vi "DAQ-WriteArray.vi"(4 "DAQ?":bool, 5 "Control Array":dbl[](array[numeric]), 6 "Limites":T2, 7 "#samples":u32, 8 "DAQ Device IN":T1={"DAQ Fs (S/s)"=10000.0, "task"="", "error"={"status"=FALSE, "code"=0, "source"=""}, "Min Value"=-10.0, "Max Value"=10.0}) -> (0 "Waveform Graph":waveform(dbl)(graph), 3 "DAQ Device OUT":T1={"DAQ Fs (S/s)"=0.0, "task"="", "error"={"status"=FALSE, "code"=0, "source"=""}, "Min Value"=-10.0, "Max Value"=10.0})   [LabVIEW 2010]
uses:
  <vilib>/DAQmx/write.llb/DAQmx Write (Analog Wfm 1Chan NSamp).vi
  <vilib>/daqmx/miscellaneous.llb/DAQmx Fill In Error Info.vi
panel:
  out "#samples 2":u32
  out "#samples out":u32
  out "Waveform":waveform(dbl)
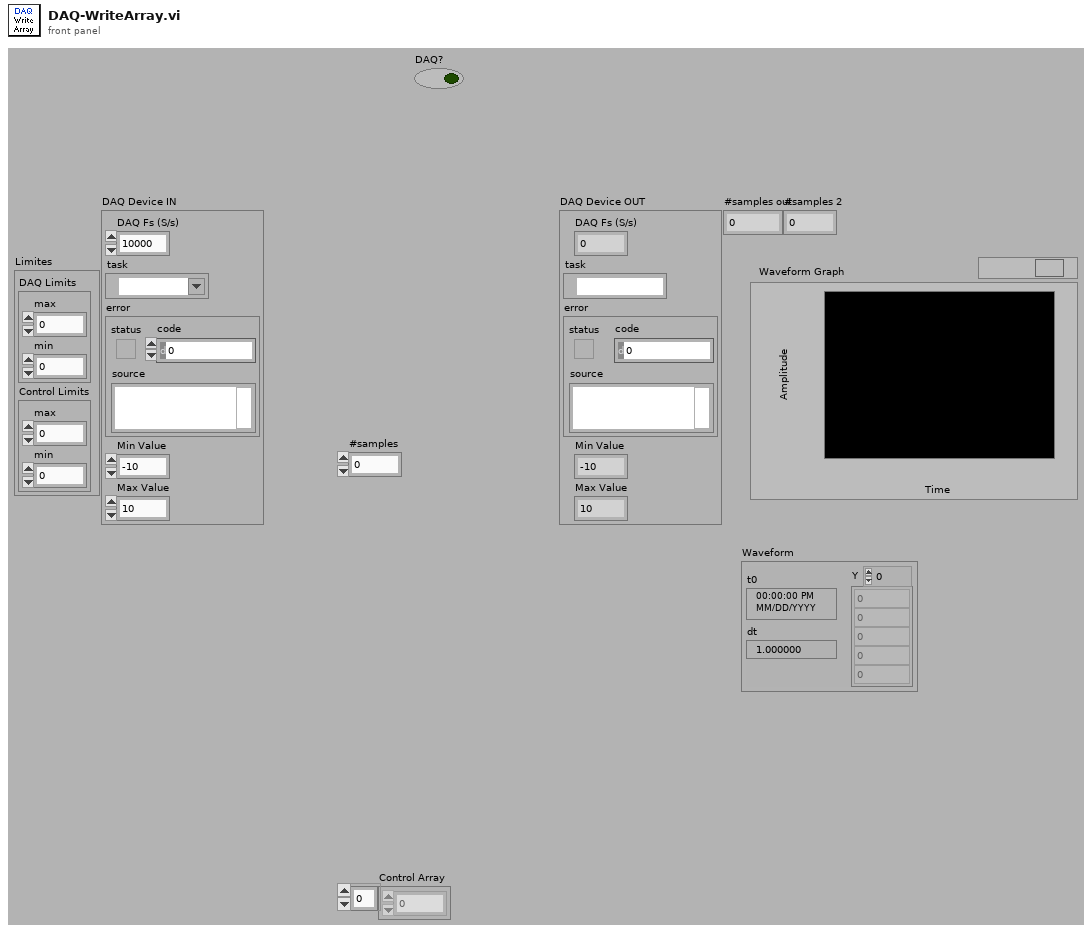
[diagram p1: front panel]
types:
  T1 = cluster{"DAQ Fs (S/s)":dbl, "task":refnum<k21>, "error":errorcluster, "Min Value":dbl, "Max Value":dbl}
  T2 = cluster{"DAQ Limits":cluster{"max":dbl, "min":dbl}, "Control Limits":cluster{"max":dbl, "min":dbl}}
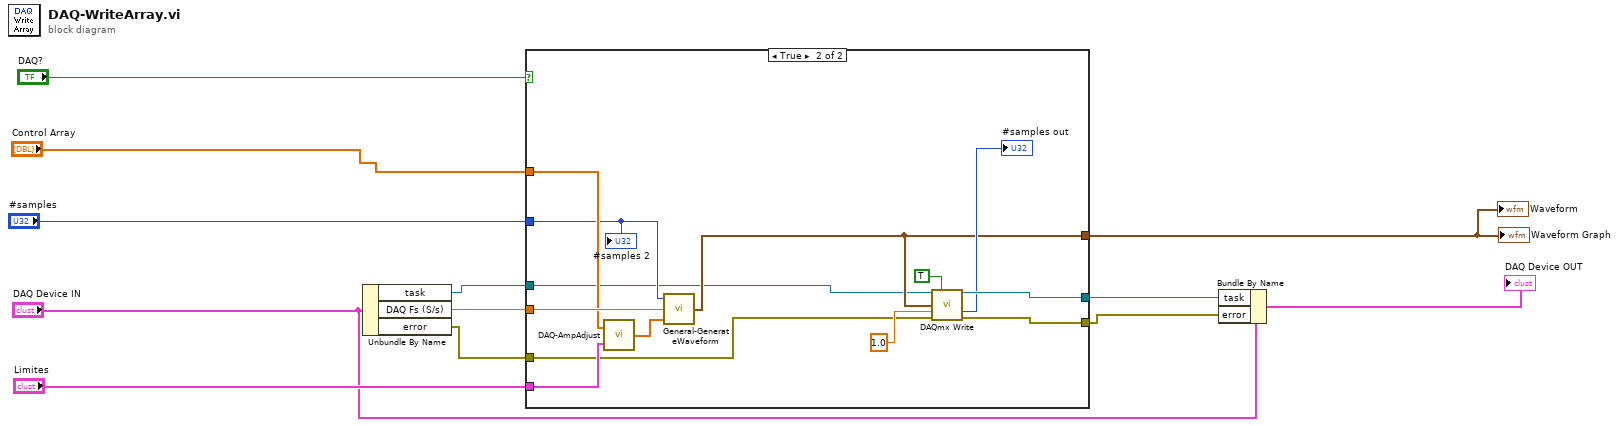
[diagram p0: block diagram]
diagram:
  n1 = Unbundle By Name("DAQ Device IN") -> ("task"=w5:refnum<k21>, "DAQ Fs (S/s)"=w1:dbl, "error"=w2:errorcluster)
  n2 = case shown="True" "DAQ?" {
    tunnel: w5 -> [w13 w16]
    tunnel: [w13 w23] -> w3
    tunnel: w2 -> [w14 w15]
    tunnel: [w14 w22] -> w4
    tunnel: w1 -> [_ w26]
    tunnel: "Control Array" -> [_ w24]
    tunnel: "#samples" -> [_ w18]
    tunnel: [_ w17] -> w10
    tunnel: "Limites" -> [_ w25]
    frame False {
    }
    frame True {
      n3 = call "DAQ-AmpAdjust.vi"("Limites"=w25, "Control Input"=w24) -> ("DAQ Output"=w27:dbl[])
      n4 = call "General-GenerateWaveform.vi"("Array"=w27, "Fs (S/s)"=w26, "#samples"=w18) -> ("Waveform"=w17:waveform(dbl))
      n5 = call-poly <vilib>:"DAQmx Write.vi"("task/channels in"=w16, "auto start"=TRUE, "data"=w17, "timeout"=1.0, "error in"=w15) -> ("task out"=w23:refnum<k21>, "number of samples written per channel"=→"#samples out":u32, "error out"=w22:errorcluster)  [unwired: 8 in]
      "#samples 2" <- w18
    }
  }
  "Waveform" <- w10
  "Waveform Graph" <- w10
  n6 = Bundle By Name(cluster="DAQ Device IN", "task"=w3, "error"=w4) -> (→"DAQ Device OUT":T1)
